vi "Read Sender.vi"(11 "Update Pump State Msg in":refnum<class "Update Pump State Msg.lvclass">) -> (2 "Sender":refnum<class "Sender.lvclass">)   [LabVIEW 2025, in "Update Pump State Msg.lvlib" / "Update Pump State Msg.lvclass"]
uses:
  Update Pump State Msg.lvclass
  <vilib>/Nathan Davis/jettl/jettl/jettl/Sender/Sender/Sender.lvclass
  Update Pump State Msg.lvclass/Update Pump State Msg.ctl
panel:
  # "This front panel should not be manipulated."
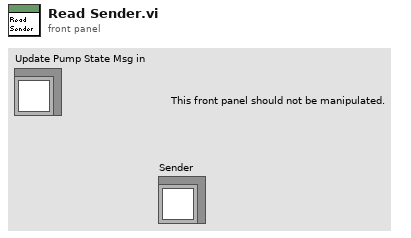
[diagram p1: front panel]
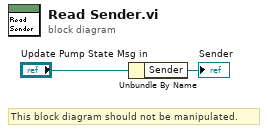
[diagram p0: block diagram]
diagram:
  # "This block diagram should not be manipulated."
  n1 = Unbundle By Name("Update Pump State Msg in") -> ("Sender"=→"Sender":refnum<class "Sender.lvclass">)
